vi "CASE1.vi"() -> ()   [LabVIEW 2020]
panel:
  out "RESPUESTA":dbl
  in  "y":dbl
  in  "x":dbl
  in  "SUMA\n\n\nRESTA":bool
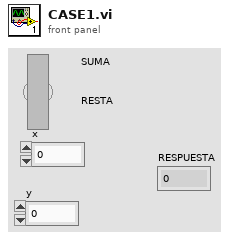
[diagram p1: front panel]
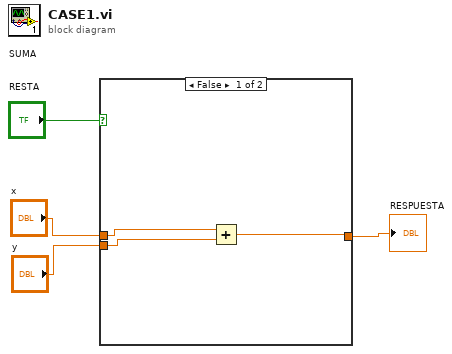
[diagram p0: block diagram]
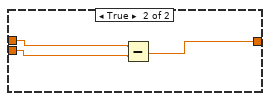
[diagram p2: hidden frame]
diagram:
  n1 = case shown="False" "SUMA\n\n\nRESTA" {
    tunnel: "y" -> [w6 w9]
    tunnel: "x" -> [w7 w10]
    tunnel: [w5 w8] -> w1
    frame False {
      n2 = Add(x=w7, y=w6) -> (x+y=w5:dbl)
    }
    frame True {
      n3 = Subtract(x=w10, y=w9) -> (x-y=w8:dbl)
    }
  }
  "RESPUESTA" <- w1
